vi "AutomatedStart.vi"() -> ()   [LabVIEW 2014]
uses:
  <vilib>/userdefined/High Color/nirio_resource_hc.ctl
  TriggerChannel.ctl
  <vilib>/FPGAPlugInAG/PCI-7813R/niLvFpga_Open_PCI-7813R.vi
  <vilib>/rvi/interface/nirviOpenFPGA/nirviOpenFPGA.xnode
  FPGA Bitfiles/W7XBolo2017_FPGATarget_fmain2014_DACRangeVoltage.lvbitx
  f_main_2014.vi
  <vilib>/rvi/interface/nirviMethod/nirviMethod.xnode
  <vilib>/FPGAPlugInAG/PCI-7813R/niLvFpga_Reset_PCI-7813R.vi
panel:
  out "Operation Watchdog":bool
  out "No. of Software Triggers \ndetected":dbl
  out "No. of Hardware Triggers \ndetected":dbl
  out "Autmated Start Loop Counter \n(Increasing every 1s)":i32
  out "Timeout ? \n(1s-10s?)":bool
  out "Hardware Trigger \ndetected":bool
  in  "Software Trigger\n(Switch until released)":bool
  in  "Stopp Button":bool
  # "Automated Start W7-X Bolometer DAQ"
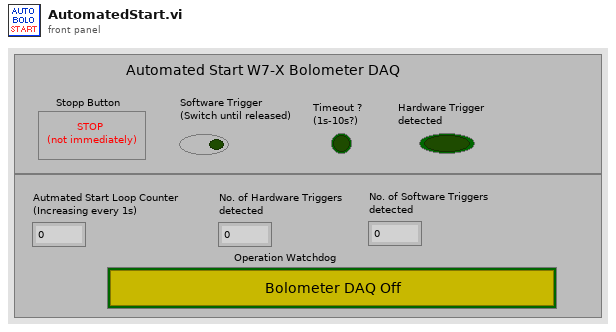
[diagram p1: front panel]
types:
  T1 = typedef "TriggerChannel.ctl" = enum16{"board0 (broken)", "board1 (t = -60sec)", "board2 (t = 0sec)"}
  T2 = enum32{"Invalid", "Standard", "Closed", "Hidden", "Minimized", "Maximized"}
  T3 = typedef "nirio_resource_hc.ctl" = tag
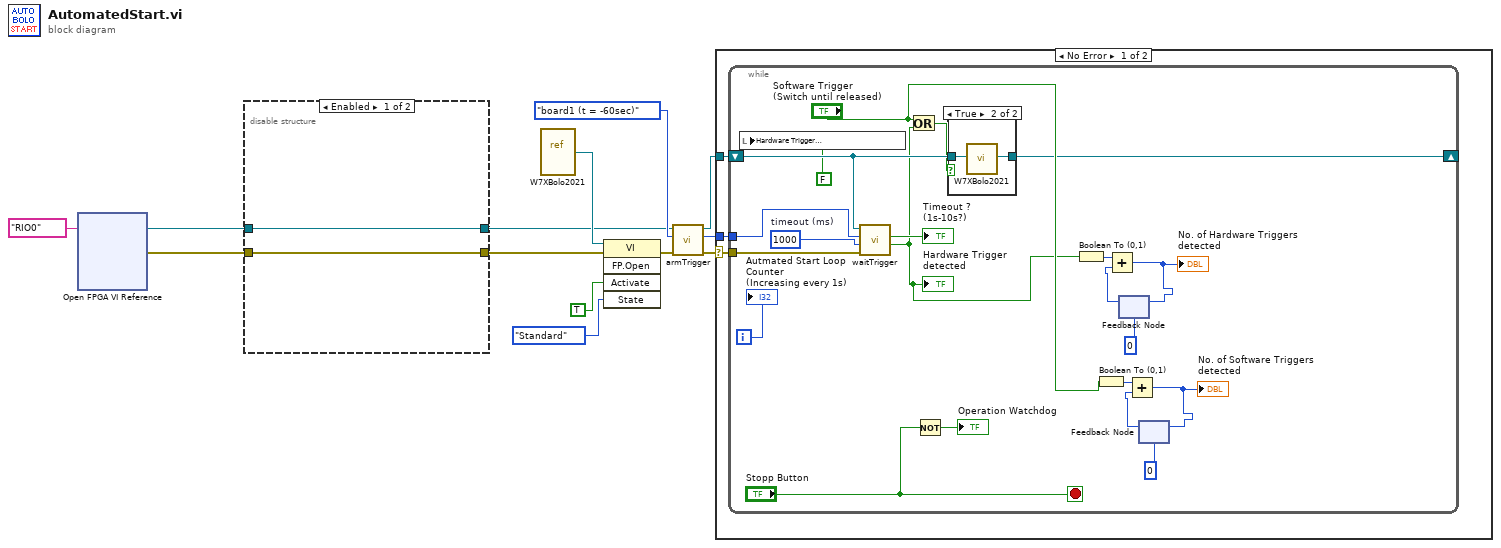
[diagram p0: block diagram]
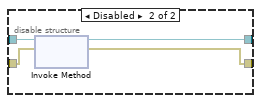
[diagram p2: hidden frame]
diagram:
  n1 = xnode "Open FPGA VI Reference"("resource name"=T3 "RIO0") -> ("FPGA VI Reference Out"=w3:refnum<k20>, "error out"=w1:errorcluster)  [unwired: 1 in]
  n2 = disable-structure shown="Enabled" {
    disable-tunnel: [w15 w17] -> w4
    disable-tunnel: w3 -> [w15 w19]
    disable-tunnel: w1 -> [w14 w18]
    disable-tunnel: [w14 w16] -> w2
    frame Enabled {
    }
    frame Disabled {
      n3 = xnode "Invoke Method"("FPGA VI Reference In"=w19, "error in"=w18) -> ("FPGA VI Reference Out"=w17:refnum<k20>, "error out"=w16:errorcluster)
    }
  }
  n4 = vi-ref "W7XBolo2021.vi"() -> (w5:refnum<vi>)
  n5 = invoke class="VI" method="FP.Open"(reference=w5, error in=w2, "Activate"=TRUE ("Activate?"), "State"=T2."Standard") -> (error out=w10:errorcluster)  [unwired: 1 in, 4 out]
  n6 = call "armTrigger.vi"("error in (no error)"=w10, "Trigger default: board0 (t = 0)"=TriggerChannel."board1 (t = -60sec)", "Refnum in"=w4) -> ("error out"=w9:errorcluster, "IRQ"=w6:i32, "Refnum out"=w7:refnum<k20>)  [unwired: 6 in]
  n7 = case shown="No Error" w9 {
    selector: w9 -> [w20 _]
    tunnel: w7 -> [w22 _]
    tunnel: w6 -> [w21 _]
    frame No Error {
      n8 = while {
        tunnel: w21 -> [w41]
        tunnel: w20 -> [w40]
        shift-right: [w23] -> _
        shift-left: w22 -> [w43]
        i -> [w37]
        stop <- "Stopp Button" stop-if-true
        w42 = 1000  # timeout (ms)
        n9 = local write "Hardware Trigger \ndetected"(FALSE) -> ()
        n10 = call "waitTrigger.vi"("error in (no error)"=w40, "timeout (ms) default: 10s"=w42, "IRQ"=w41, "Refnum in"=w43) -> ("Boolean"=w26:bool, "Timed Out"=→"Timeout ? \n(1s-10s?)":bool)  [unwired: 4 in, 2 out]
        "Hardware Trigger \ndetected" <- w26
        n11 = Or(x="Software Trigger\n(Switch until released)", y=w26) -> (x .or. y?=w32:bool)
        n12 = Not(x="Stopp Button") -> (.not. x?=→"Operation Watchdog":bool)
        n13 = case shown="True" w32 {
          tunnel: w43 -> [w44 w46]
          tunnel: [w44 w45] -> w23
          frame False {
          }
          frame True {
            n14 = call "W7XBolo2021.vi"("FPGA VI\nReference In"=w46) -> ("FPGA VI Reference Out"=w45:refnum<k20>)
          }
        }
        n15 = Boolean To (0,1)(Boolean=w26) -> (0, 1=w35:i16)
        n16 = Boolean To (0,1)(Boolean="Software Trigger\n(Switch until released)") -> (0, 1=w30:i16)
        n17 = feedback #1(i16 0) -> (w36:i16)
        n18 = Add(x=w35, y=w36) -> (x+y=w33:i16)
        "No. of Hardware Triggers \ndetected" <- w33
        n19 = feedback-in #1(w33) -> ()
        n20 = feedback #2(i16 0) -> (w31:i16)
        n21 = Add(x=w30, y=w31) -> (x+y=w28:i16)
        "No. of Software Triggers \ndetected" <- w28
        n22 = feedback-in #2(w28) -> ()
        "Autmated Start Loop Counter \n(Increasing every 1s)" <- w37
      }
    }
    frame Error {
    }
  }
